vi "ReadRemoteControl.vi"(8 "Error In":errorcluster, 11 "reference in":refnum<class "Button.lvclass">) -> (0 "Error Out":errorcluster, 2 "RemoteControl":refnum<class "RemoteControl.lvclass">, 3 "reference out":refnum<class "Button.lvclass">)   [LabVIEW 2024, in "Button.lvclass"]
uses:
  Button.lvclass
  Button.lvclass/Button.ctl
  Invoker/RemoteControl_class/RemoteControl.lvclass
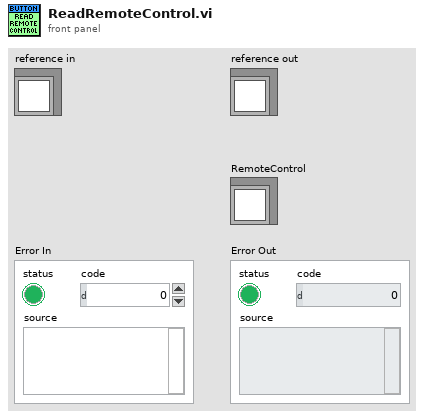
[diagram p1: front panel]
types:
  T1 = typedef "Button.lvclass/ObjectAttributes.ctl" = cluster{"RemoteControl":refnum<class "RemoteControl.lvclass">}
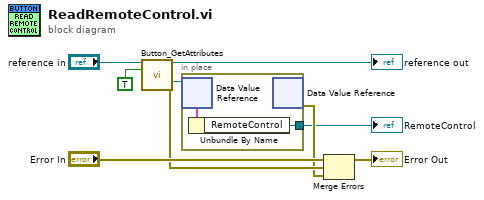
[diagram p0: block diagram]
diagram:
  n1 = call "Button_GetAttributes.vi"("reference in"="reference in", "OnlyGetDvrReference(False)"=TRUE) -> ("reference out"=→"reference out":refnum<class "Button.lvclass">, "DataRef"=w2:refnum<data-value>, "Error Out"=w8:errorcluster)  [unwired: 10 in, 1 out]
  n2 = in-place {
    in-place-border: [w11] -> w1
    n3 = in-place-dvr #1(w2) -> (w10:T1)  [unwired: 1 out]
    n4 = Unbundle By Name(w10) -> ("RemoteControl"=w11:refnum<class "RemoteControl.lvclass">)
    n5 = in-place-dvr #1() -> (w6:errorcluster)  [unwired: 1 in, 1 out]
  }
  "RemoteControl" <- w1
  n6 = Merge Errors("Error In", w8, w6) -> (→"Error Out":errorcluster)
